vi "set line pattern start finish with follow me.vi"() -> ()   [LabVIEW 2021]
uses:
  <userlib>/Nanonis Prog Interface V5/Scan/Grid/LinePatternSet.vi
  <userlib>/Nanonis Prog Interface V5/Nanonis Prog Interface.lvlib
panel:
  in  "line position":enum16{"start", "finish"}(ring)
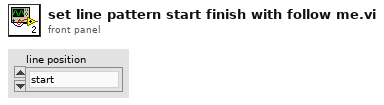
[diagram p1: front panel]
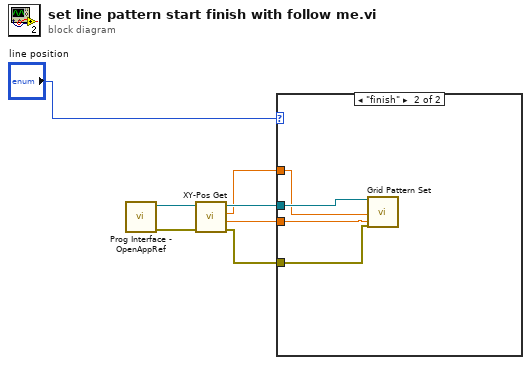
[diagram p0: block diagram]
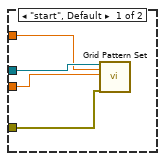
[diagram p2: hidden frame]
diagram:
  n1 = call <userlib>:"Prog Interface - OpenAppRef.vi"() -> ("Error out"=w6:errorcluster, "Application reference"=w7:refnum<vi>)  [unwired: 6 in]
  n2 = call <userlib>:"XY-Pos Get.vi"("error in (no error)"=w6, "Application ref in"=w7) -> ("error out"=w4:errorcluster, "Y (m)"=w2:sgl, "X (m)"=w3:sgl, "Application ref out"=w5:refnum<vi>)  [unwired: 5 in]
  n3 = case shown="\"finish\"" "line position" {
    tunnel: w5 -> [w11 w15]
    tunnel: w4 -> [w10 w14]
    tunnel: w3 -> [w9 w13]
    tunnel: w2 -> [w8 w12]
    frame "start", Default {
      n4 = call-poly <userlib>:"Grid Pattern Set.vi"("Application ref in"=w11, "Start X1 (m) (NaN=no change)"=w9, "Start Y1 (m) (NaN=no change)"=w8, "error in (no error)"=w10) -> ()  [unwired: 14 in, 2 out]
    }
    frame "finish" {
      n5 = call-poly <userlib>:"Grid Pattern Set.vi"("Application ref in"=w15, "End X2 (m) (NaN=no change)"=w13, "End Y2 (m) (NaN=no change)"=w12, "error in (no error)"=w14) -> ()  [unwired: 14 in, 2 out]
    }
  }
